vi "Read Data.vi"(8 "error in":errorcluster, 11 "Modbus in":refnum<class "Modbus.lvclass">) -> (0 "error out":errorcluster, 2 "Data Read":string, 3 "Modbus out":refnum<class "Modbus.lvclass">)   [LabVIEW 2021, in "Modbus.lvclass"]
uses:
  Modbus.lvclass
  Modbus.lvclass/Modbus.ctl
  <vilib>/NI/Modbus Library/API/Master/Modbus Master.lvclass
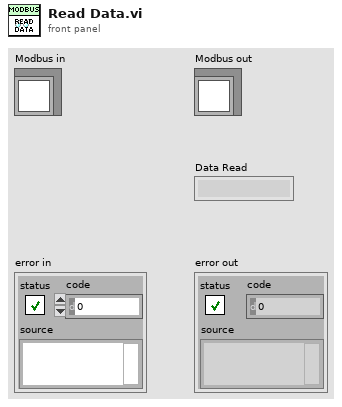
[diagram p1: front panel]
types:
  T1 = enum16{"big-endian, network order", "native, host order", "little-endian"}
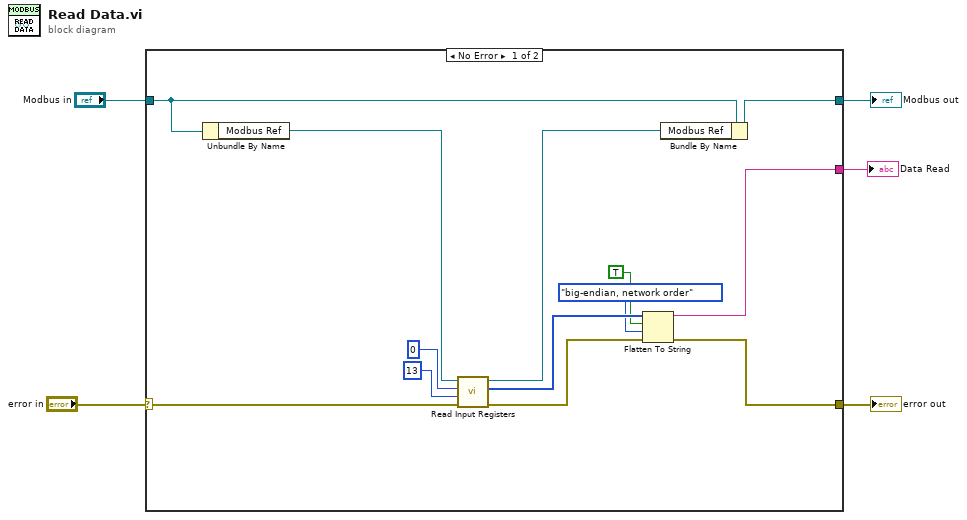
[diagram p0: block diagram]
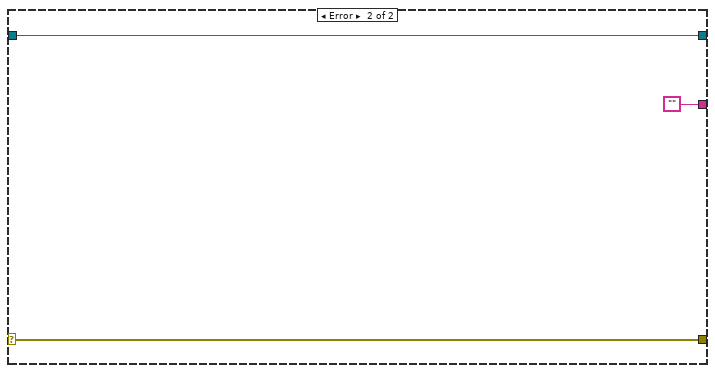
[diagram p2: hidden frame]
diagram:
  n1 = case shown="No Error" "error in" {
    selector: "error in" -> [w18 w20]
    tunnel: "Modbus in" -> [w17 w21]
    tunnel: [w13 w21] -> w4
    tunnel: [w7 w20] -> w2
    tunnel: [w6 ""] -> w1
    frame No Error {
      n2 = Unbundle By Name(w17) -> ("Modbus Ref"=w16:refnum<class "Modbus Master.lvclass">)
      n3 = call-dynamic "Read Input Registers.vi"("error in"=w18, "number of inputs"=u16 13, "starting address"=u16 0, "Modbus master in"=w16) -> ("error out"=w8:errorcluster, "register values"=w11:u16[], "Modbus master out"=w12:refnum<class "Modbus Master.lvclass">)  [unwired: 5 in]
      n4 = Flatten To String(anything=w11, prepend array or string size? (T)=TRUE, byte order (0:big-endian, network order)=T1."big-endian, network order", error in (no error)=w8) -> (data string=w6:string, error out=w7:errorcluster)  [unwired: 1 out]
      n5 = Bundle By Name(cluster=w17, "Modbus Ref"=w12) -> (w13:refnum<class "Modbus.lvclass">)
    }
    frame Error {
    }
  }
  "error out" <- w2
  "Modbus out" <- w4
  "Data Read" <- w1
